vi "Assemble Module.vi"() -> ()   [LabVIEW 2016]
uses:
  Classes/Assembly/Database Assembly/Database Assembly.lvclass
  Classes/Controller/Controller.lvclass
panel:
  in  "Control":cluster{"Component ID":dbl}
  in  "Assembly Queue":cluster{}
  in  "Add step to Assembly":bool
  in  "Step Number":dbl
  in  "Module Settings":T1(array[cluster])
  in  "Stop":bool
  in  "Go":bool
  in  "Assembly Tray Number":dbl
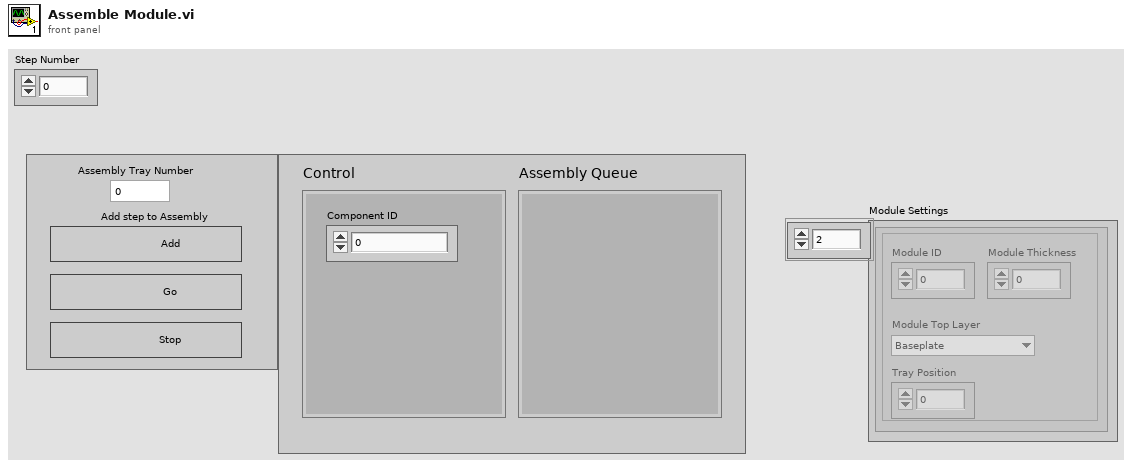
[diagram p1: front panel]
types:
  T1 = cluster{"Module ID":dbl, "Module Thickness":dbl, "Module Top Layer":enum16{"Baseplate", "Kapton", "Sensor", "PCB"}, "Tray Position":dbl}[]
  T2 = typedef "Controller.lvclass/Controllers.ctl" = cluster{"I-O.lvclass":refnum<class "I-O.lvclass">, "Motion.lvclass":refnum<class "Motion.lvclass">, "Dispenser.lvclass":refnum<class "Dispenser.lvclass">}
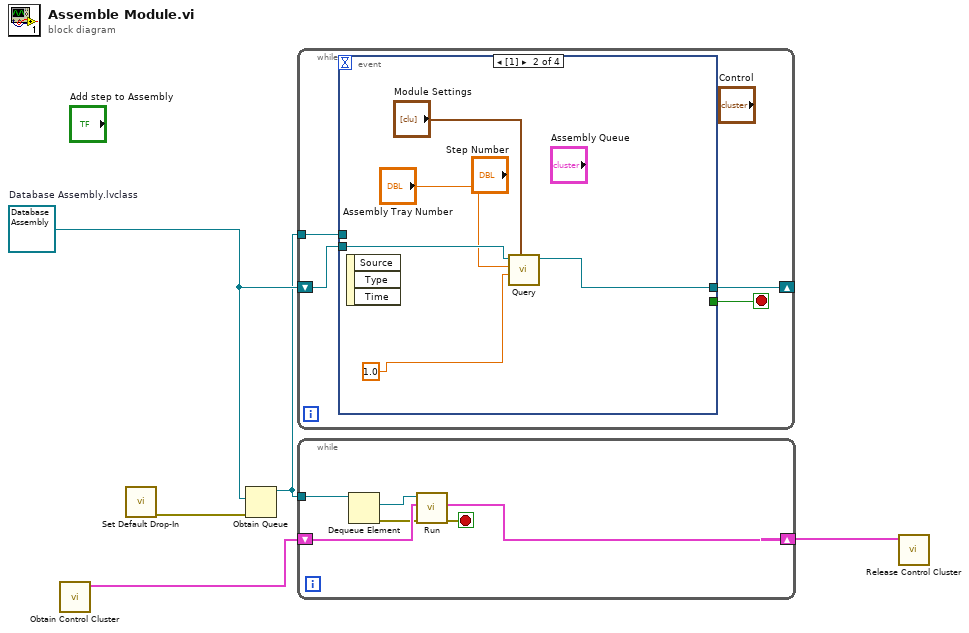
[diagram p0: block diagram]
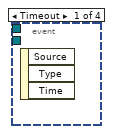
[diagram p2: hidden frame]
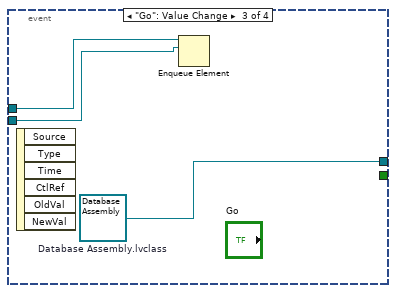
[diagram p3: hidden frame]
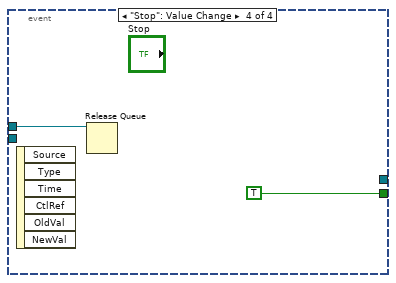
[diagram p4: hidden frame]
diagram:
  w5 = refnum<class "Database Assembly.lvclass"> refnum  # Database Assembly.lvclass
  n1 = call "Obtain Control Cluster.vi"() -> ("Control Out"=w3:T2)  [unwired: 11 in]
  n2 = call "Set Default Drop-In.vi"() -> ("error out"=w1:errorcluster)  [unwired: 11 in]
  n3 = Obtain Queue(element data type=w5, error in (no error)=w1) -> (queue out=w4:refnum<queue>)  [unwired: 3 in, 2 out]
  n4 = while {
    shift-right: [w8] -> _
    shift-left: w5 -> [w9]
    tunnel: w4 -> [w7]
    stop <- w6 stop-if-true
    n5 = event shown="[1]" {
      selector: _ -> [_ _ _ _]
      dyn-events: _ -> [_ _ _ _]
      timeout: _ -> [_ _ _ _]
      tunnel: w9 -> [_ w14 w15 _]
      tunnel: [_ w13 w16 _] -> w8
      tunnel: w7 -> [_ _ w17 w19]
      tunnel: [_ _ _ TRUE] -> w6
      event Timeout {
        n6 = event-data() -> ()  [unwired: 1 in, 3 out]
      }
      event #1 (no event record) {
        n7 = event-data() -> ()  [unwired: 1 in, 3 out]
        n8 = call "Query.vi"("Module Settings"="Module Settings", "Region"=1.0, "Tray"="Assembly Tray Number", "Database Assembly in"=w14) -> ("Database Assembly out"=w13:refnum<class "Database Assembly.lvclass">)  [unwired: 6 in, 1 out]
      }
      event "Go": Value Change {
        w16 = refnum<class "Database Assembly.lvclass"> refnum  # Database Assembly.lvclass
        n9 = event-data() -> ()  [unwired: 1 in, 6 out]
        n10 = Enqueue Element(queue=w17, element=w15) -> ()  [unwired: 2 in, 3 out]
      }
      event "Stop": Value Change {
        n11 = event-data() -> ()  [unwired: 1 in, 6 out]
        n12 = Release Queue(queue=w19) -> ()  [unwired: 2 in, 3 out]
      }
    }
  }
  n13 = while {
    tunnel: w4 -> [w25]
    shift-right: [w21] -> w2
    shift-left: w3 -> [w24]
    stop <- w23 stop-if-true
    n14 = Dequeue Element(queue=w25) -> (element=w20:refnum<class "Database Assembly.lvclass">, error out=w22:errorcluster)  [unwired: 2 in, 2 out]
    n15 = call-dynamic "Run.vi"("error in (no error)"=w22, "Control In"=w24, "Assembly In"=w20) -> ("error out"=w23:errorcluster, "Control Out"=w21:T2)  [unwired: 6 in, 1 out]
  }
  n16 = call "Release Control Cluster.vi"("output cluster"=w2) -> ()  [unwired: 11 in]
